vi "CheckWallState.vi"(0 "Position":dbl[](array[numeric]), 1 "Field":refnum<class "Field.lvclass">, 5 "error in (no error)":errorcluster) -> (14 "WallState":T1=enum."FrontWall", 19 "error out":errorcluster)   [LabVIEW 2024, in "DefendAreaTactic.lvclass"]
uses:
  DefendAreaTactic.lvclass
  WallPositions.ctl
  Field_class/Field.lvclass
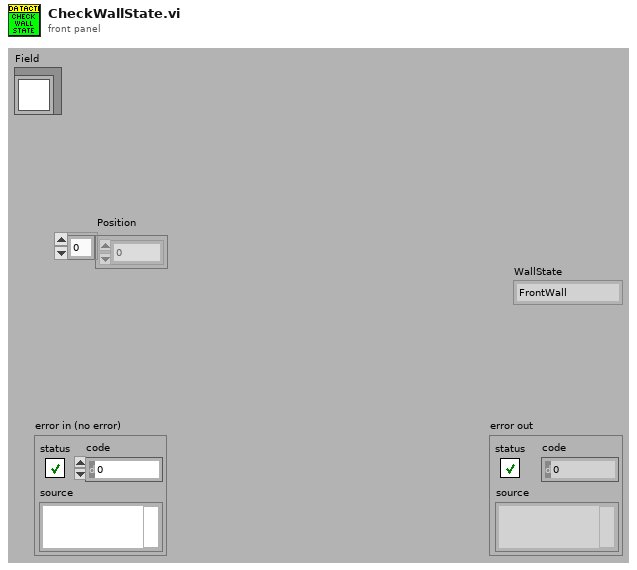
[diagram p1: front panel]
types:
  T1 = typedef "WallPositions.ctl" = enum16{"LeftWall", "LeftCorner", "FrontWall", "RightCorner", "RightWall"}
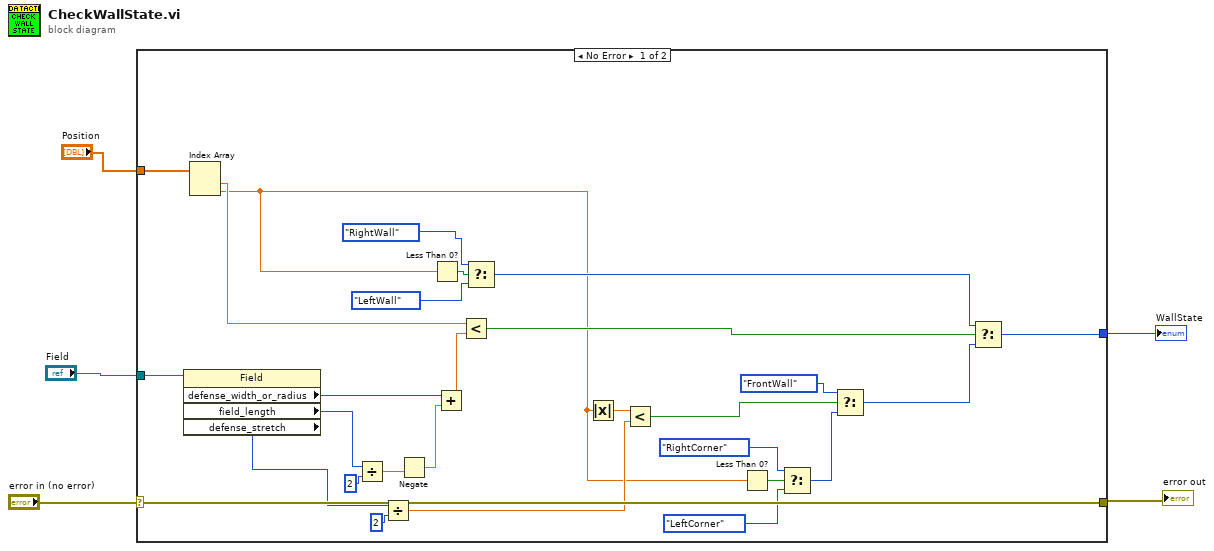
[diagram p0: block diagram]
diagram:
  n1 = case shown="No Error" "error in (no error)" {
    selector: "error in (no error)" -> [w33 w34]
    tunnel: [w33 w34] -> w4
    tunnel: "Field" -> [w32 _]
    tunnel: "Position" -> [w31 _]
    tunnel: [w7 _] -> w1
    frame No Error {
      n2 = property class="Field"(reference=w32) -> ("defense_width_or_radius"=w27:i32, "field_length"=w30:i32, "defense_stretch"=w15:i32)  [unwired: 1 in, 2 out]
      n3 = Index Array(array=w31) -> (element #1=w24:dbl, element #2=w10:dbl)  [unwired: 2 in]
      n4 = Divide(x=w30, y=2) -> (x/y=w28:dbl)
      n5 = Divide(x=w15, y=2) -> (x/y=w14:dbl)
      n6 = Negate(x=w28) -> (-x=w26:dbl)
      n7 = Less Than 0?(x=w10) -> (x < 0?=w22:bool)
      n8 = Add(x=w27, y=w26) -> (x+y=w25:dbl)
      n9 = Less?(x=w24, y=w25) -> (x < y?=w23:bool)
      n10 = Select(t=WallPositions."RightWall", s=w22, f=WallPositions."LeftWall") -> (s? t:f=w21:T1)
      n11 = Absolute Value(x=w10) -> (abs(x)=w18:dbl)
      n12 = Less?(x=w18, y=w14) -> (x < y?=w17:bool)
      n13 = Less Than 0?(x=w10) -> (x < 0?=w11:bool)
      n14 = Select(t=WallPositions."RightCorner", s=w11, f=WallPositions."LeftCorner") -> (s? t:f=w12:T1)
      n15 = Select(t=WallPositions."FrontWall", s=w17, f=w12) -> (s? t:f=w13:T1)
      n16 = Select(t=w21, s=w23, f=w13) -> (s? t:f=w7:T1)
    }
    frame Error {
    }
  }
  "error out" <- w4
  "WallState" <- w1
